vi "Main.vi"() -> ()   [LabVIEW 2010]
uses:
  DLL-s/MakeFullImmitationStepDLL/Release/MakeFullImmitationStepDLL.dll
panel:
  out "CA STATES":string[][](array[string])
  out "CA PROCESSES":string[](array[string])=["Инициализация", "ОстановВсехПроцессовИстартПроцИнициализация", "КонтрольДостоверности", "КонтрольДостоверностиОткрытияЗатвораВакуумного", "КонтрольДостоверностиОткрЗатВакуумного", "КонтрольДостоверностиЗакрЗатВакуумного", "КонтрольДостоверностиСостоянияСапуна", "КонтрольДостоверностиСостоянияУстройстваПлавПуска", "КонтрольДостоверностиСостоянияПитанияВакуумногоНасоса", "КонтрольДостоверностиСостоянияПитанияВентилятора", "КонтрольДостоверностиСостоянияПитанияРегТемпературы", "КонтрольДостоверностиСостоянияПитанияРегУровня", "КонтрольДостоверностиУровняВодыМинимум", "КонтрольДостоверностиУровняВодыМаксимум", "КонтрольДостоверностиСостоянияПитанияНасОхлаждения", "ЧтениеФактПараметров_с_Датчиков", "РЕГУЛЯТОР_ТРАФИКА", "ЧтениеКольцевогоБуфера", "ОбработкаКомандИзмененияНП_от_ГУИ", "ОбработкаКомандУправления_от_ГУИ", "КонтрольИзменения_ФП_P_ВбакеКомпрессора", "КонтрольИзменения_ФП_P_Впатрубке", "КонтрольИзменения_ФП_T_Врубашке", "КонтрольИзменения_ФП_T_Вбаке", "КонтрольИзменения_ФП_P_ВтрубеСидер", "КонтрольВеличиныОткачкиВауумнойТрубыСидеростата", "КонтрольГотовностиВакуума_в_Вакуумной_Трубе", "КонтрольУровняВодыБакаОхлаждения", "КонтрольТемпературыВодыБакаОхлаждения", "КонтрольТемпературыРубашкиОхлаждения", "КонтрольДавленияВбакеКомпрессора", "ВКЛ_ПИТ_ВЕНТИЛЯТОР", "ВЫК_ПИТ_ВЕНТИЛЯТОР", "КонтрольСостоянияПитанияВентилятора", "КонтрольСпонтанногоВыключенияВентилятора", "КонтрольСпонтанногоВключенияВентилятора", "КонтрольСостоянияЗатвораВакуумного", "ОТКР_ЗАТВОР_ВАК", "ЗАКР_ЗАТВОР_ВАК", "КонтрольСпонтанногоЗакрытияЗатвораВакуумного", "КонтрольСпонтанногоОткрытияЗатвораВакуумного", "ОТКР_САПУН", "ЗАКР_САПУН", "КонтрольСостоянияПитанияСапуна", "КонтрольСпонтанногоЗакрытияСапуна", "КонтрольСпонтанногоОткрытияСапуна", "ВКЛ_ПИТ_ВАК_НАСОСА", "ВЫК_ПИТ_ВАК_НАСОСА", "КонтрольСостоянияПитанияВакуумногоНасоса", "КонтрольСпонтанногоВыключенияВакНасоса", "КонтрольСпонтанногоВключенияВакНасоса", "ВКЛ_ПИТ_РЕГ_Т", "ВЫК_ПИТ_РЕГ_Т", "КонтрольСостоянияПитанияРЕГ_Т", "КонтрольСпонтанногоВыключенияРЕГ_Т", "КонтрольСпонтанногоВключенияРЕГ_Т", "ВКЛ_ПИТ_РЕГ_УР", "ВЫК_ПИТ_РЕГ_УР", "КонтрольСостоянияПитанияРЕГ_УР", "КонтрольСпонтанногоВыключенияРЕГ_УР", "КонтрольСпонтанногоВключенияРЕГ_УР", "ВКЛ_ПИТ_НАС_ОХЛ", "ВЫК_ПИТ_НАС_ОХЛ", "КонтрольСостоянияПитанияНАС_ОХЛ", "КонтрольСпонтанногоВыключенияНасосаОхлаждения", "КонтрольСпонтанногоВключенияНасосаОхлаждения", "ВКЛ_УСТР_ПЛАВ_ПУСКА", "ВЫК_УСТР_ПЛАВ_ПУСКА", "КонтрольСостоянияПитанияПЛАВ_ПУСКА", "КонтрольСпонтанногоВыключенияПлавнПуска", "КонтрольСпонтанногоВключенияПлавнПуска", "ВКЛ_ВАКУУМИРОВАНИЕ_ТРУБЫ", "ВЫК_ВАКУУМИРОВАНИЕ_ТРУБЫ", "ВКЛ_ВАКУУМНУЮ_ПОДСИСТЕМУ", "ВЫК_ВАКУУМНУЮ_ПОДСИСТЕМУ"]
  out "CA DESCR":T1
  out "VP DESCR":T2
  out "VM DESCR":T3
  out "exists":bool
  out "appended array":i32[](array[numeric])
  out "Scalar":bool
  out "Проект":path
  out "Stop Ver Button":bool
  in  "Pause":bool
  out "Верификация запущена":bool
  in  "max queue size (-1, unlimited)":i32
  out "error":i32
  in  "verifier2scenariousControlOutMsgs":cluster{"MSG":i16, "param":i32, "Type":i16}[](array[cluster])
  out "Verification":bool
  in  "scenarioStates":cluster{"TimeInState":u16, "cur_state":i8}[](array[cluster])
  in  "verStates":cluster{"TimeInState":u16, "cur_state":i8}[](array[cluster])
  in  "vplantStates":cluster{"TimeInState":u16, "cur_state":i8}[](array[cluster])
  in  "algStates":cluster{"TimeInState":u16, "cur_state":i8}[](array[cluster])
  in  "virtualPlant2GUIOutputMsgs":cluster{"MSG":i16, "param":i32, "Type":i16}[](array[cluster])
  in  "verifier2GUIOutputMsgs":cluster{"MSG":i16, "param":i32, "Type":i16}[](array[cluster])
  in  "algOutputMsgs":cluster{"MSG":i16, "param":i32, "Type":i16}[](array[cluster])
  in  "scenarios2VerifierOutputMsgs":cluster{"MSG":i16, "param":i32, "Type":i16}[](array[cluster])
  in  "scenarios2VirtPlantOutputMsgs":cluster{"MSG":i16, "param":i32, "Type":i16}[](array[cluster])
  in  "Cluster":cluster{"MSG":i16, "param":i32, "Type":i16}
  in  "scenarios2AlgOutputMsgs":cluster{"MSG":i16, "param":i32, "Type":i16}[](array[cluster])
  in  "algOutputPorts":i8[](array[numeric])
  in  "algInputPorts":i8[](array[numeric])
  in  "TEST MODE":bool
  out "DLLDriverReference":refnum<vi> caption="CA vi reference"
  in  "Open editor":bool
  in  "START Button":bool
  out "VB vi reference":refnum<vi> caption="CA vi reference"
  out "SCB vi reference":refnum<vi> caption="CA vi reference"
  out "VP vi reference":refnum<vi> caption="CA vi reference"
  out "CA vi reference":refnum<vi>
  out "error out":errorcluster
  in  "Открыть панель БВ":bool
  in  "Открыть панель БУС":bool
  in  "Открыть панель АУ":bool
  in  "stop":bool
  in  "Открыть панель ВОУ":bool
  out "Автоматический режим работы":bool
  in  "Режим работы:":bool
  # "Ручной"
  # "Автоматический"
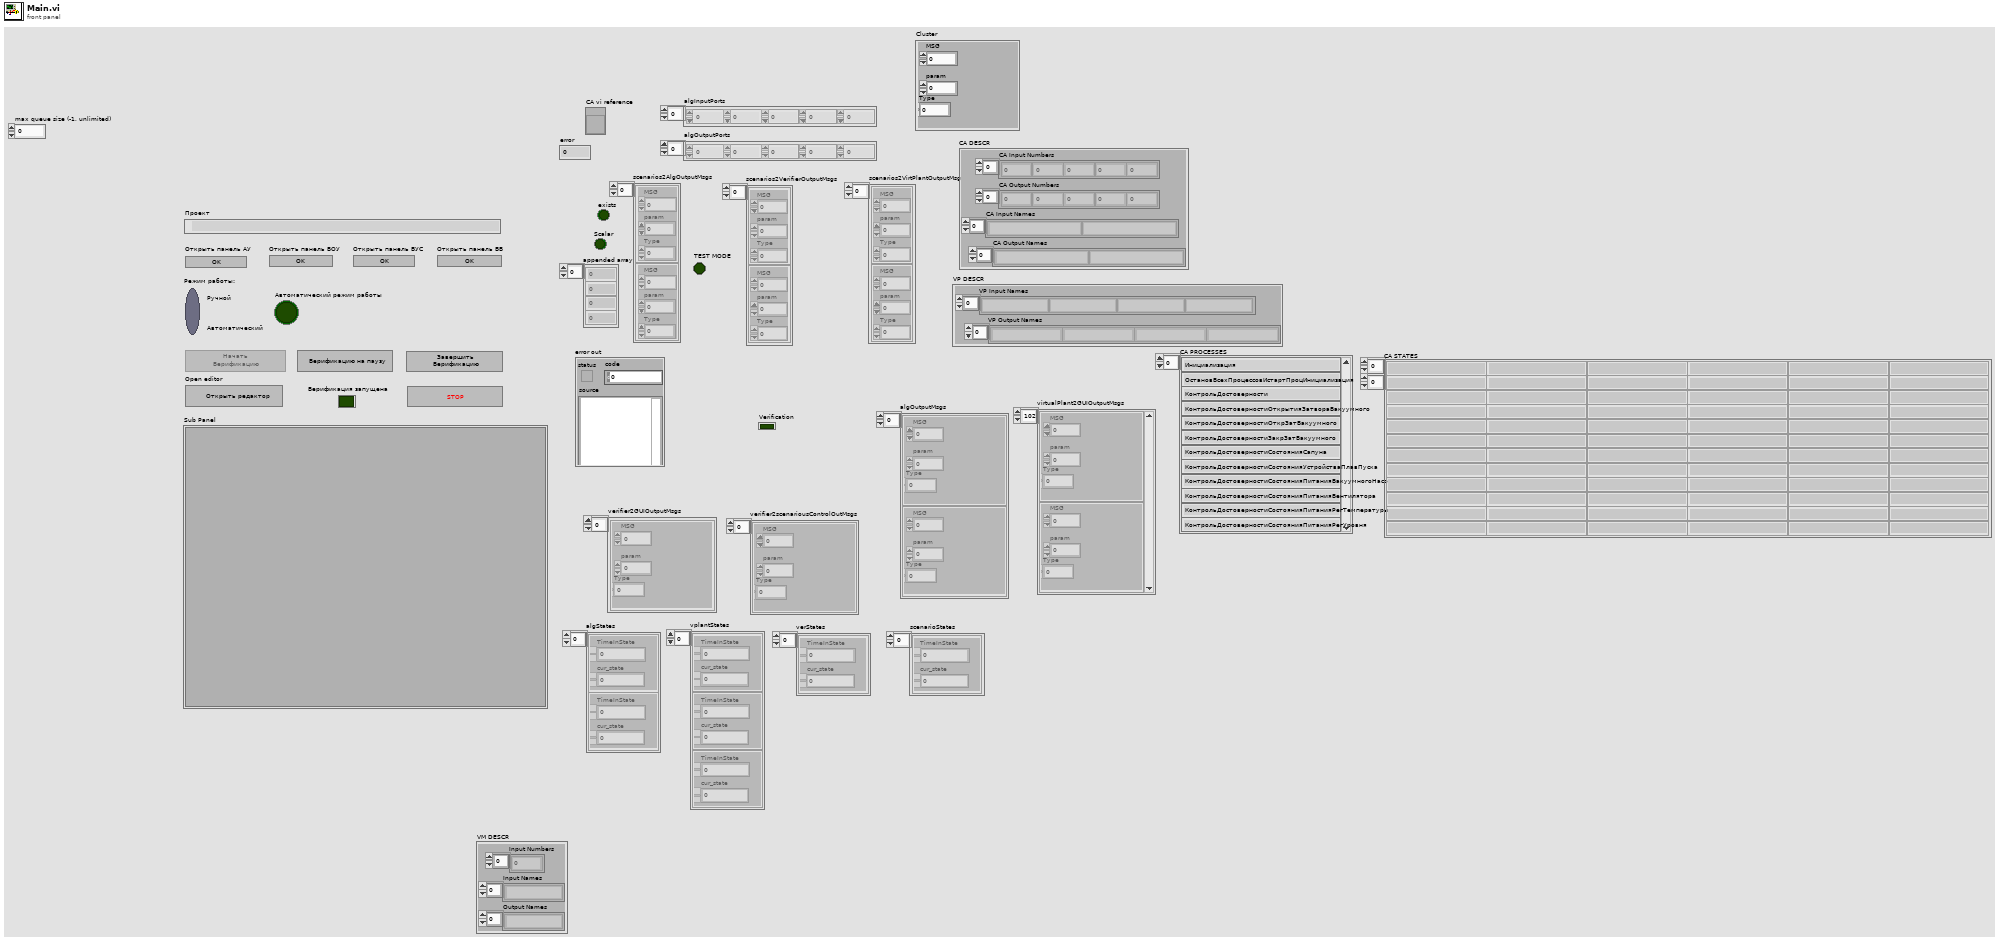
[diagram p1: front panel]
types:
  T1 = cluster{"CA Input Numbers":i32[], "CA Output Numbers ":i32[], "CA Input Names":string[], "CA Output Names ":string[]}
  T2 = cluster{"VP Input Names":string[], "VP Output Names ":string[]}
  T3 = cluster{"Input Numbers":i32[], "Input Names":string[], "Output Names ":string[]}
  T4 = enum8{"Enabled", "Disabled", "Disabled and Grayed Out"}
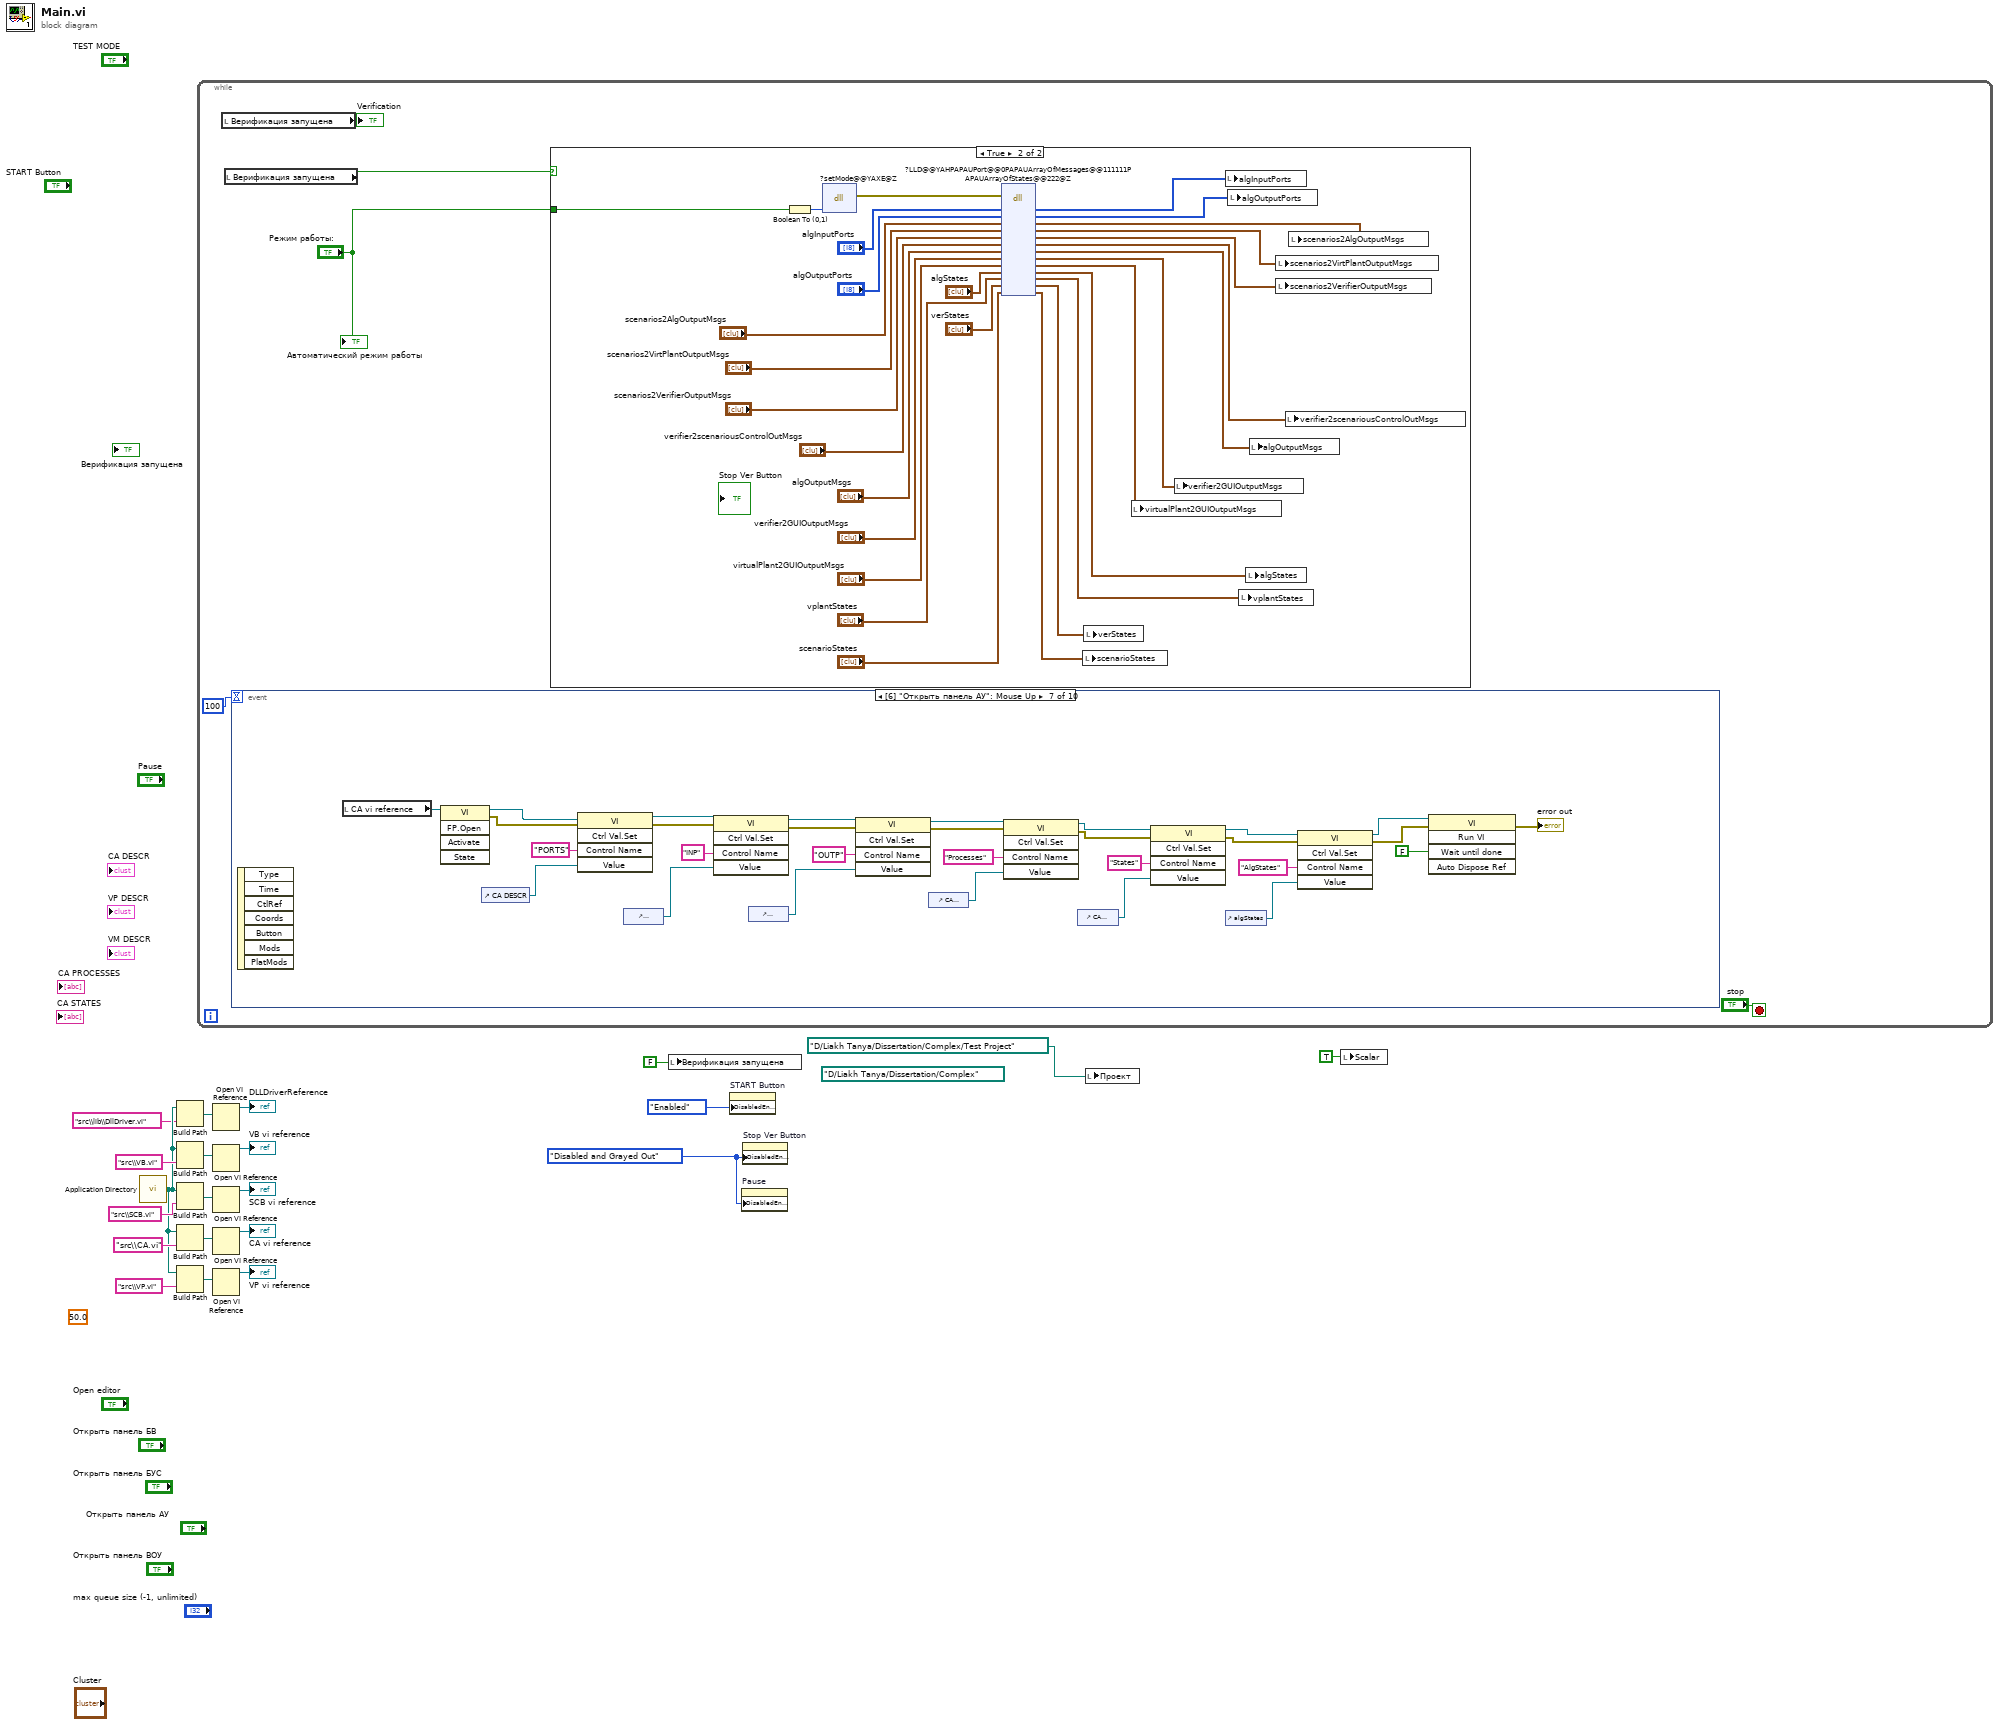
[diagram p0: block diagram]
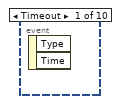
[diagram p3: hidden frame]
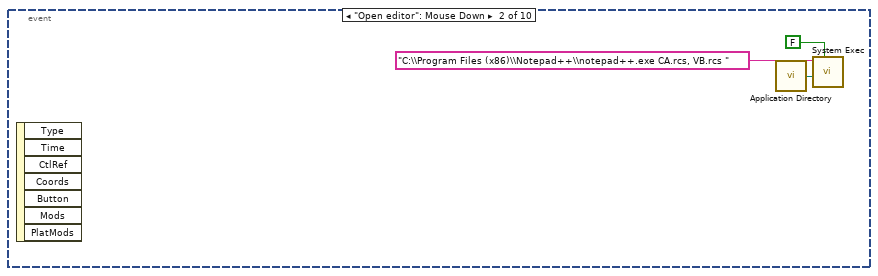
[diagram p4: hidden frame]
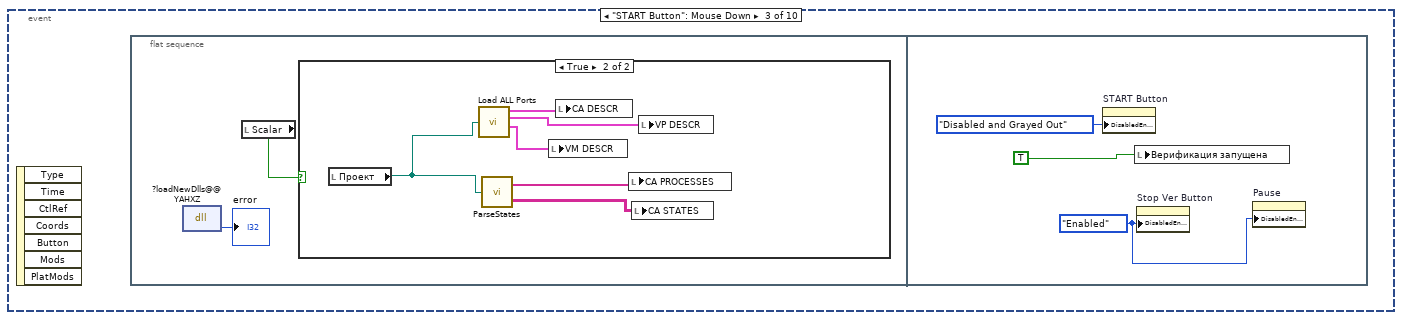
[diagram p5: hidden frame]
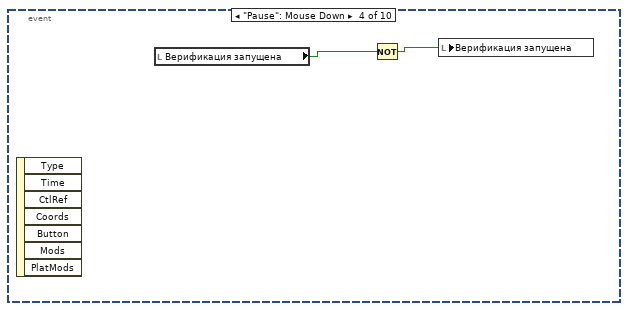
[diagram p7: hidden frame]
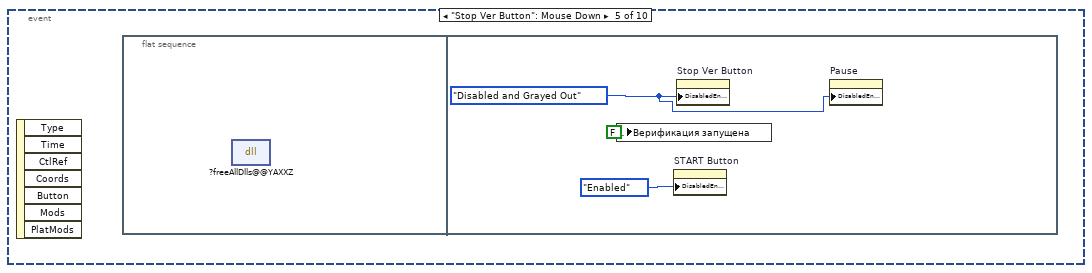
[diagram p8: hidden frame]
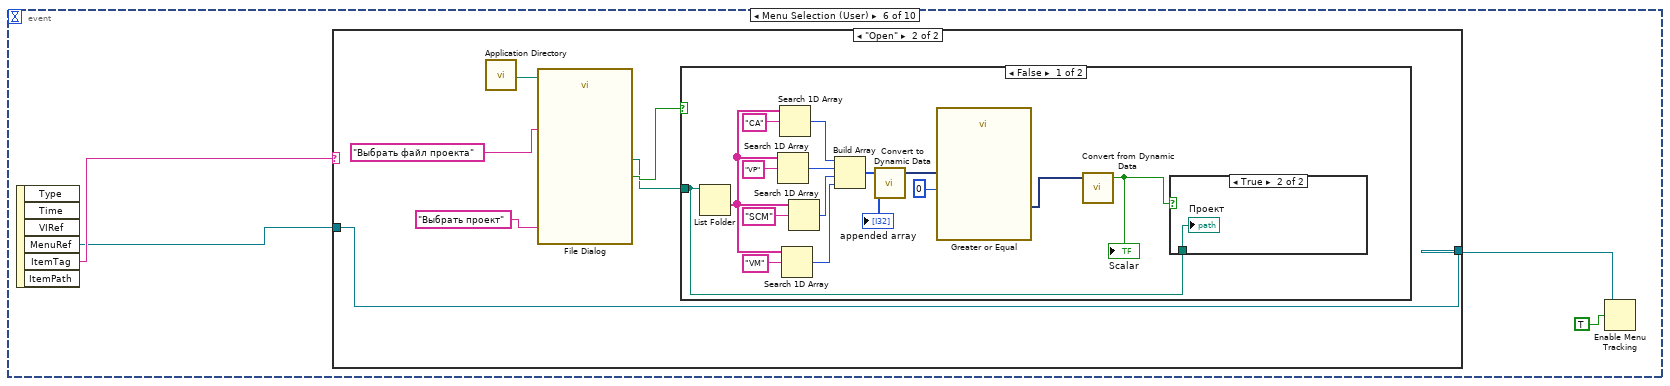
[diagram p9: hidden frame]
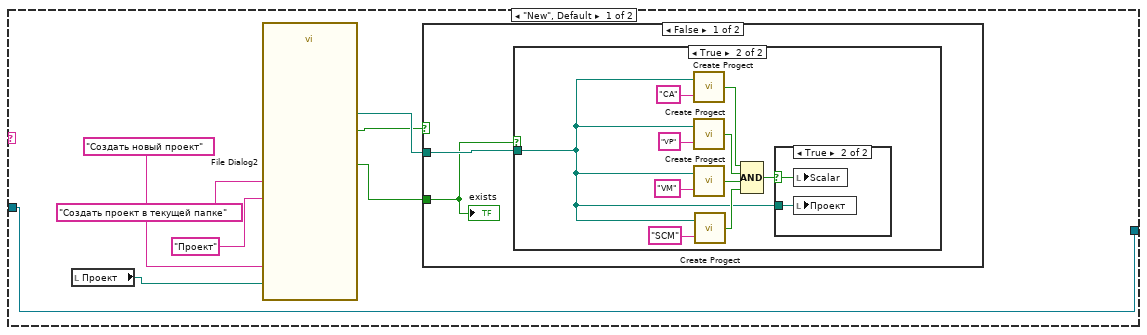
[diagram p10: hidden frame]
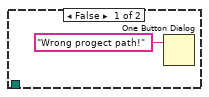
[diagram p14: hidden frame]
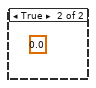
[diagram p15: hidden frame]
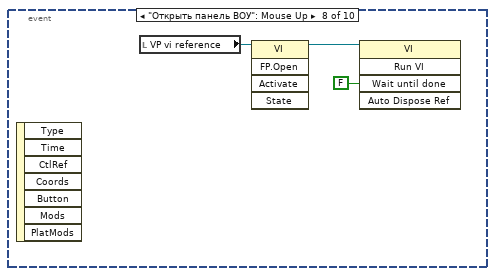
[diagram p16: hidden frame]
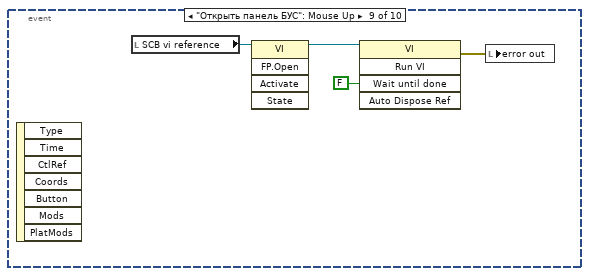
[diagram p17: hidden frame]
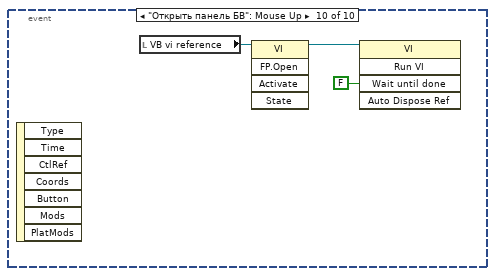
[diagram p18: hidden frame]
diagram:
  (unwired) path "D:/Liakh Tanya/Dissertation/Complex" ("Проект")
  w3 = T4."Disabled and Grayed Out" ("Disabled")
  (unwired) 50.0 ("Gauge")
  n1 = call <vilib>:"Application Directory.vi"() -> ("Application Directory"=w7:path)
  n2 = Build Path(base path=w7, name or relative path="src\\lib\\DllDriver.vi") -> (appended path=w8:path)
  n3 = Build Path(base path=w7, name or relative path="src\\VB.vi") -> (appended path=w13:path)
  n4 = Build Path(base path=w7, name or relative path="src\\SCB.vi") -> (appended path=w16:path)
  n5 = Build Path(base path=w7, name or relative path="src\\CA.vi") -> (appended path=w21:path)
  n6 = Build Path(base path=w7, name or relative path="src\\VP.vi") -> (appended path=w18:path)
  n7 = while {
    stop <- "stop" stop-if-true
    n8 = local read "Верификация запущена"() -> (→"Verification":bool)
    n9 = local read "Верификация запущена"() -> (w24:bool)
    n10 = event shown="[6] \"Открыть панель АУ\": Mouse Up" {
      selector: _ -> [_ _ _ _ _ _ _ _ _ _]
      dyn-events: _ -> [_ _ _ _ _ _ _ _ _ _]
      timeout: 100 -> [_ _ _ _ _ _ _ _ _ _]
      event Timeout {
        n11 = event-data() -> ()  [unwired: 1 in, 2 out]
      }
      event "Open editor": Mouse Down {
        n12 = event-data() -> ()  [unwired: 1 in, 7 out]
        n13 = call <vilib>:"Application Directory.vi"() -> ("Application Directory"=w56:path)
        n14 = call <vilib>:"System Exec.vi"("wait until completion? (T)"=FALSE, "working directory"=w56, "command line"="C:\\Program Files (x86)\\Notepad++\\notepad++.exe CA.rcs, VB.rcs ") -> ()  [unwired: 5 in, 4 out]
      }
      event "START Button": Mouse Down {
        n15 = event-data() -> ()  [unwired: 1 in, 7 out]
        n16 = flat-sequence {
          frame #0 {
            n17 = dll-call lib="D:/Liakh Tanya/Dissertation/Complex/DLL-s/MakeFullImmitationStepDLL/Release/MakeFullImmitationStepDLL.dll" fn="?loadNewDlls@@YAHXZ" label="Load NEW DLLs"() -> ("error"=→"error":i32)  [unwired: 3 in, 2 out]
            n18 = local read "Scalar"() -> (w59:bool)
            n19 = case shown="True" w59 {
              frame False {
              }
              frame True {
                n20 = local read "Проект"() -> (w63:path)
                n21 = call "Load ALL Ports.vi"("path"=w63) -> ("VM Cluster"=w64:T3, "VP Cluster"=w65:T2, "CA Cluster"=w66:T1)  [unwired: 1 out]
                n22 = call "ParseStates.vi"("base path"=w63) -> ("CA STATES"=w61:string[][], "CA PROCESSES"=w62:string[])
                n23 = local write "VM DESCR"(w64) -> ()
                n24 = local write "CA DESCR"(w66) -> ()
                n25 = local write "CA PROCESSES"(w62) -> ()
                n26 = local write "CA STATES"(w61) -> ()
                n27 = local write "VP DESCR"(w65) -> ()
              }
            }
          }
          frame #1 {
            w67 = T4."Enabled" ("Disabled")
            n28 = property on="START Button" class="Bool (strict)"("DisabledEnum"=T4."Disabled and Grayed Out" ("Disabled")) -> ()  [unwired: 2 in, 2 out]
            n29 = local write "Верификация запущена"(TRUE ("VerificationRunning")) -> ()
            n30 = property on="Stop Ver Button" class="Bool (strict)"("DisabledEnum"=w67) -> ()  [unwired: 2 in, 2 out]
            n31 = property on="Pause" class="Bool (strict)"("DisabledEnum"=w67) -> ()  [unwired: 2 in, 2 out]
          }
        }
      }
      event "Pause": Mouse Down {
        n32 = event-data() -> ()  [unwired: 1 in, 7 out]
        n33 = local read "Верификация запущена"() -> (w71:bool)
        n34 = Not(x=w71) -> (.not. x?=w70:bool)
        n35 = local write "Верификация запущена"(w70) -> ()
      }
      event "Stop Ver Button": Mouse Down {
        n36 = event-data() -> ()  [unwired: 1 in, 7 out]
        n37 = flat-sequence {
          frame #0 {
            n38 = dll-call lib="D:/Liakh Tanya/Dissertation/Complex/DLL-s/MakeFullImmitationStepDLL/Release/MakeFullImmitationStepDLL.dll" fn="?freeAllDlls@@YAXXZ" label="FREE DLLs"() -> ()  [unwired: 4 in, 2 out]
          }
          frame #1 {
            w72 = T4."Disabled and Grayed Out" ("Disabled")
            n39 = local write "Верификация запущена"(FALSE ("VerificationRunning")) -> ()
            n40 = property on="START Button" class="Bool (strict)"("DisabledEnum"=T4."Enabled" ("Disabled")) -> ()  [unwired: 2 in, 2 out]
            n41 = property on="Stop Ver Button" class="Bool (strict)"("DisabledEnum"=w72) -> ()  [unwired: 2 in, 2 out]
            n42 = property on="Pause" class="Bool (strict)"("DisabledEnum"=w72) -> ()  [unwired: 2 in, 2 out]
          }
        }
      }
      event Menu Selection (User) {
        n43 = event-data() -> ("MenuRef"=w76:refnum<k9>, "ItemTag"=w77:string)  [unwired: 1 in, 4 out]
        n44 = case shown="\"Open\"" w77 {
          tunnel: w76 -> [w86 w104]
          tunnel: [w86 w104] -> w75
          frame "New", Default {
            n45 = local read "Проект"() -> (w79:path)
            n46 = call "File Dialog2"("start path"=w79, "prompt"="Создать новый проект" ("default name"), "button label"="Создать проект в текущей папке" ("pattern label"), "default name"="Проект") -> ("selected path"=w82:path, "exists"=w81:bool, "cancelled"=w80:bool)  [unwired: 8 in, 1 out]
            n47 = case shown="False" w80 {
              tunnel: w82 -> [w88 _]
              tunnel: w81 -> [w87 _]
              frame False {
                n48 = case shown="True" w87 {
                  tunnel: w88 -> [_ w89]
                  frame False {
                  }
                  frame True {
                    n49 = call "Create Progect.vi"("element"="CA", "selected path"=w89) -> ("Boolean"=w94:bool)
                    n50 = call "Create Progect.vi"("element"="VP", "selected path"=w89) -> ("Boolean"=w93:bool)
                    n51 = call "Create Progect.vi"("element"="VM", "selected path"=w89) -> ("Boolean"=w91:bool)
                    n52 = call "Create Progect.vi"("element"="SCM", "selected path"=w89) -> ("Boolean"=w92:bool)
                    n53 = Compound Arithmetic op=AND(w94, w93, w91, w92) -> (w90:bool)
                    n54 = case shown="True" w90 {
                      selector: w90 -> [_ w100]
                      tunnel: w89 -> [_ w99]
                      frame False {
                      }
                      frame True {
                        n55 = local write "Scalar"(w100) -> ()
                        n56 = local write "Проект"(w99) -> ()
                      }
                    }
                  }
                }
                "exists" <- w87
              }
              frame True {
              }
            }
          }
          frame "Open" {
            n57 = call <vilib>:"Application Directory.vi"() -> ("Application Directory"=w105:path)
            n58 = call "File Dialog"("start path"=w105, "prompt"="Выбрать файл проекта" ("default name"), "button label"="Выбрать проект" ("pattern label")) -> ("selected path"=w101:path, "cancelled"=w102:bool)  [unwired: 9 in, 2 out]
            n59 = case shown="False" w102 {
              tunnel: w101 -> [w108 _]
              frame False {
                n60 = List Folder(path=w108) -> (folder names=w117:string[])  [unwired: 3 in, 3 out]
                n61 = Search 1D Array(1D array=w117, element="VP") -> (index of element=w114:i32)  [unwired: 1 in]
                n62 = Search 1D Array(1D array=w117, element="CA") -> (index of element=w115:i32)  [unwired: 1 in]
                n63 = Search 1D Array(1D array=w117, element="VM") -> (index of element=w112:i32)  [unwired: 1 in]
                n64 = Search 1D Array(1D array=w117, element="SCM") -> (index of element=w113:i32)  [unwired: 1 in]
                n65 = Build Array(w115, w114, w113, w112) -> (w111:i32[])
                "appended array" <- w111
                n66 = call "Convert to Dynamic Data"("Array"=w111) -> ("Dynamic Data Type"=w110:dynamicdata)  [unwired: 3 in]
                n67 = call "Greater or Equal"("Constant Value to Compare Against"=0, "Operand 1"=w110) -> ("Result"=w109:dynamicdata)  [unwired: 8 in, 1 out]
                n68 = call "Convert from Dynamic Data"("Dynamic Data Type"=w109) -> ("Scalar"=w107:bool)  [unwired: 3 in]
                "Scalar" <- w107
                n69 = case shown="True" w107 {
                  tunnel: w108 -> [_ w123]
                  frame False {
                    n70 = One Button Dialog(message="Wrong progect path!") -> ()  [unwired: 1 in, 1 out]
                  }
                  frame True {
                    "Проект" <- w123
                  }
                }
              }
              frame True {
                (unwired) 0.0
              }
            }
          }
        }
        n71 = Enable Menu Tracking(3:TRUE ("enable (T)"), 4:w75) -> ()  [unwired: 1 in, 2 out]
      }
      event "Открыть панель АУ": Mouse Up {
        n72 = event-data() -> ()  [unwired: 1 in, 7 out]
        n73 = local read "CA vi reference"() -> (w150:refnum<vi>)
        n74 = invoke class="VI" method="FP.Open"(reference=w150) -> (reference out=w149:refnum<vi>, error out=w147:errorcluster)  [unwired: 4 in, 3 out]
        n75 = control-ref of="CA DESCR"() -> (w146:refnum<vi>)
        n76 = invoke class="VI" method="Ctrl Val.Set"(reference=w149, error in=w147, "Control Name"="PORTS", "Value"=w146) -> (reference out=w145:refnum<vi>, error out=w144:errorcluster)  [unwired: 1 in, 3 out]
        n77 = control-ref of="algInputPorts"() -> (w142:refnum<vi>)
        n78 = invoke class="VI" method="Ctrl Val.Set"(reference=w145, error in=w144, "Control Name"="INP", "Value"=w142) -> (reference out=w140:refnum<vi>, error out=w139:errorcluster)  [unwired: 1 in, 3 out]
        n79 = control-ref of="algOutputPorts"() -> (w138:refnum<vi>)
        n80 = invoke class="VI" method="Ctrl Val.Set"(reference=w140, error in=w139, "Control Name"="OUTP", "Value"=w138) -> (reference out=w135:refnum<vi>, error out=w134:errorcluster)  [unwired: 1 in, 3 out]
        n81 = control-ref of="CA PROCESSES"() -> (w126:refnum<vi>)
        n82 = invoke class="VI" method="Ctrl Val.Set"(reference=w135, error in=w134, "Control Name"="Processes", "Value"=w126) -> (reference out=w133:refnum<vi>, error out=w132:errorcluster)  [unwired: 1 in, 3 out]
        n83 = control-ref of="CA STATES"() -> (w125:refnum<vi>)
        n84 = invoke class="VI" method="Ctrl Val.Set"(reference=w133, error in=w132, "Control Name"="States", "Value"=w125) -> (reference out=w130:refnum<vi>, error out=w129:errorcluster)  [unwired: 1 in, 3 out]
        n85 = control-ref of="algStates"() -> (w124:refnum<vi>)
        n86 = invoke class="VI" method="Ctrl Val.Set"(reference=w130, error in=w129, "Control Name"="AlgStates", "Value"=w124) -> (reference out=w128:refnum<vi>, error out=w127:errorcluster)  [unwired: 1 in, 3 out]
        n87 = invoke class="VI" method="Run VI"(reference=w128, error in=w127, "Wait until done"=FALSE ("Wait Until Done")) -> (error out=→"error out":errorcluster)  [unwired: 2 in, 4 out]
      }
      event "Открыть панель ВОУ": Mouse Up {
        n88 = event-data() -> ()  [unwired: 1 in, 7 out]
        n89 = local read "VP vi reference"() -> (w153:refnum<vi>)
        n90 = invoke class="VI" method="FP.Open"(reference=w153) -> (reference out=w154:refnum<vi>)  [unwired: 4 in, 4 out]
        n91 = invoke class="VI" method="Run VI"(reference=w154, "Wait until done"=FALSE ("Wait Until Done")) -> ()  [unwired: 3 in, 5 out]
      }
      event "Открыть панель БУС": Mouse Up {
        n92 = event-data() -> ()  [unwired: 1 in, 7 out]
        n93 = local read "SCB vi reference"() -> (w157:refnum<vi>)
        n94 = invoke class="VI" method="FP.Open"(reference=w157) -> (reference out=w158:refnum<vi>)  [unwired: 4 in, 4 out]
        n95 = invoke class="VI" method="Run VI"(reference=w158, "Wait until done"=FALSE ("Wait Until Done")) -> (error out=w156:errorcluster)  [unwired: 3 in, 4 out]
        n96 = local write "error out"(w156) -> ()
      }
      event "Открыть панель БВ": Mouse Up {
        n97 = event-data() -> ()  [unwired: 1 in, 7 out]
        n98 = local read "VB vi reference"() -> (w160:refnum<vi>)
        n99 = invoke class="VI" method="FP.Open"(reference=w160) -> (reference out=w161:refnum<vi>)  [unwired: 4 in, 4 out]
        n100 = invoke class="VI" method="Run VI"(reference=w161, "Wait until done"=FALSE ("Wait Until Done")) -> ()  [unwired: 3 in, 5 out]
      }
    }
    n101 = case shown="True" w24 {
      tunnel: "Режим работы:" -> [_ w55]
      frame False {
      }
      frame True {
        n102 = Boolean To (0,1)(Boolean=w55) -> (0, 1=w54:i16)
        n103 = dll-call lib="D:/Liakh Tanya/Dissertation/Complex/DLL-s/MakeFullImmitationStepDLL/Release/MakeFullImmitationStepDLL.dll" fn="?setMode@@YAXE@Z" label="setMode"("mode"=w54) -> (error out=w53:errorcluster)  [unwired: 5 in, 1 out]
        n104 = dll-call lib="D:/Liakh Tanya/Dissertation/Complex/DLL-s/MakeFullImmitationStepDLL/Release/MakeFullImmitationStepDLL.dll" fn="?LLD@@YAHPAPAUPort@@0PAPAUArrayOfMessages@@111111PAPAUArrayOfStates@@222@Z" label="Init"(error in=w53, "algInputPorts"="algInputPorts", "algOutputPorts"="algOutputPorts", "scenarios2AlgOutputMsgs"="scenarios2AlgOutputMsgs", "scenarios2VirtPlantOutputMsgs"="scenarios2VirtPlantOutputMsgs", "scenarios2VerifierOutputMsgs"="scenarios2VerifierOutputMsgs", "verifier2scenariousControlOutMsgs,"="verifier2scenariousControlOutMsgs", "algOutputMsgs"="algOutputMsgs", "verifier2GUIOutputMsgs"="verifier2GUIOutputMsgs", "virtualPlant2GUIOutputMsgs"="virtualPlant2GUIOutputMsgs", "algStates"="algStates", "vplantStates"="vplantStates", "verStates"="verStates", "scenarioStates"="scenarioStates") -> ("algInputPorts"=w39:i8[], "algOutputPorts"=w37:i8[], "scenarios2AlgOutputMsgs"=w33:cluster{"MSG":i16, "param":i32, "Type":i16}[], "scenarios2VirtPlantOutputMsgs"=w31:cluster{"MSG":i16, "param":i32, "Type":i16}[], "scenarios2VerifierOutputMsgs"=w32:cluster{"MSG":i16, "param":i32, "Type":i16}[], "verifier2scenariousControlOutMsgs,"=w29:cluster{"MSG":i16, "param":i32, "Type":i16}[], "algOutputMsgs"=w36:cluster{"MSG":i16, "param":i32, "Type":i16}[], "verifier2GUIOutputMsgs"=w27:cluster{"MSG":i16, "param":i32, "Type":i16}[], "virtualPlant2GUIOutputMsgs"=w35:cluster{"MSG":i16, "param":i32, "Type":i16}[], "algStates"=w38:cluster{"TimeInState":u16, "cur_state":i8}[], "vplantStates"=w34:cluster{"TimeInState":u16, "cur_state":i8}[], "verStates"=w28:cluster{"TimeInState":u16, "cur_state":i8}[], "scenarioStates"=w30:cluster{"TimeInState":u16, "cur_state":i8}[])  [unwired: 3 in, 2 out]
        n105 = local write "scenarioStates"(w30) -> ()
        n106 = local write "verStates"(w28) -> ()
        n107 = local write "virtualPlant2GUIOutputMsgs"(w35) -> ()
        n108 = local write "verifier2GUIOutputMsgs"(w27) -> ()
        n109 = local write "algInputPorts"(w39) -> ()
        n110 = local write "algOutputPorts"(w37) -> ()
        n111 = local write "vplantStates"(w34) -> ()
        n112 = local write "algStates"(w38) -> ()
        n113 = local write "algOutputMsgs"(w36) -> ()
        n114 = local write "scenarios2VirtPlantOutputMsgs"(w31) -> ()
        n115 = local write "scenarios2VerifierOutputMsgs"(w32) -> ()
        n116 = local write "verifier2scenariousControlOutMsgs"(w29) -> ()
        n117 = local write "scenarios2AlgOutputMsgs"(w33) -> ()
      }
    }
    "Автоматический режим работы" <- "Режим работы:"
  }
  n118 = Open VI Reference(vi path=w8) -> (vi reference=→"DLLDriverReference":refnum<vi>)  [unwired: 5 in, 1 out]
  n119 = Open VI Reference(vi path=w13) -> (vi reference=→"VB vi reference":refnum<vi>)  [unwired: 5 in, 1 out]
  n120 = Open VI Reference(vi path=w16) -> (vi reference=→"SCB vi reference":refnum<vi>)  [unwired: 5 in, 1 out]
  n121 = Open VI Reference(vi path=w21) -> (vi reference=→"CA vi reference":refnum<vi>)  [unwired: 5 in, 1 out]
  n122 = Open VI Reference(vi path=w18) -> (vi reference=→"VP vi reference":refnum<vi>)  [unwired: 5 in, 1 out]
  n123 = local write "Верификация запущена"(FALSE ("VerificationRunning")) -> ()
  n124 = property on="START Button" class="Bool (strict)"("DisabledEnum"=T4."Enabled" ("Disabled")) -> ()  [unwired: 2 in, 2 out]
  n125 = property on="Pause" class="Bool (strict)"("DisabledEnum"=w3) -> ()  [unwired: 2 in, 2 out]
  n126 = property on="Stop Ver Button" class="Bool (strict)"("DisabledEnum"=w3) -> ()  [unwired: 2 in, 2 out]
  n127 = local write "Проект"(path "D:/Liakh Tanya/Dissertation/Complex/Test Project" ("Проект")) -> ()
  n128 = local write "Scalar"(TRUE ("Scalar")) -> ()
